vi "InitDrive.vi"   [LabVIEW 2018]
uses:
  <vilib>/Rock Robotics/WPI/ThirdParty/REV Robotics/SPARK MAX/Typedef/Spark MAX Idle Mode.ctl
  refnums.vi
  <vilib>/Rock Robotics/WPI/MotorControl/WPI_MotorControlOpen SPARK_MAX.vi
  <vilib>/Rock Robotics/SystemInterfaces/DIO/FPGA_DIOPWMChannel.ctl
types:
  T1 = typedef "Spark MAX Idle Mode.ctl" = enum16{"Coast", "Brake"}
  T2 = typedef "FPGA_DIOPWMChannel.ctl" = enum8{"PWM 0", "PWM 1", "PWM 2", "PWM 3", "PWM 4", "PWM 5", "PWM 6", "PWM 7", "PWM 8", "PWM 9", "PWM MXP 0", "PWM MXP 1", "PWM MXP 2", "PWM MXP 3", "PWM MXP 4", "PWM MXP 5", "PWM MXP 6", "PWM MXP 7", "PWM MXP 8", "PWM MXP 9", "Invalid"}
  T3 = typedef "WPI_MotorControlDeviceRef.ctl" = cluster{"DeviceStatus":errorcluster, "Type":T4, "PWM":cluster{"PWM Channel":T2, "DeadBand":T5}, "CAN":cluster{"Device Number":u8, "SetOutput VI Ref":variant, "GetOutput VI Ref":variant, "Enable VI Ref":variant, "Disable VI Ref":variant, "Data":variant}, "Invert":bool, "DIO PWM":cluster{"PWM \"Enable\" Channel":T2, "DIOChannel":T6, "PWM Rate":dbl}}
  T4 = typedef "WPI_MotorControlType.ctl" = enum16{"PWM", "CAN", "DIO PWM"}
  T5 = typedef "WPI_PWMDeadband.ctl" = cluster{"Name":string, "maxPositivePwm":i32, "minPositivePwm":i32, "centerPwm":i32, "maxNegativePwm":i32, "minNegativePwm":i32, "angularRange":u16}
  T6 = typedef "FPGA_DIOChannel.ctl" = enum8{"DIO 0", "DIO 1", "DIO 2", "DIO 3", "DIO 4", "DIO 5", "DIO 6", "DIO 7", "DIO 8", "DIO 9", "DIO MXP 0", "DIO MXP 1", "DIO MXP 2", "DIO MXP 3", "DIO MXP 4", "DIO MXP 5", "DIO MXP 6", "DIO MXP 7", "DIO MXP 8", "DIO MXP 9", "DIO MXP 10", "DIO MXP 11", "DIO MXP 12", "DIO MXP 13", "DIO MXP 14", "DIO MXP 15", "SPI Port CS1", "SPI Port CS2", "SPI Port CS3", "SPI Port MISO", "SPI Port MOSI", "Invalid"}
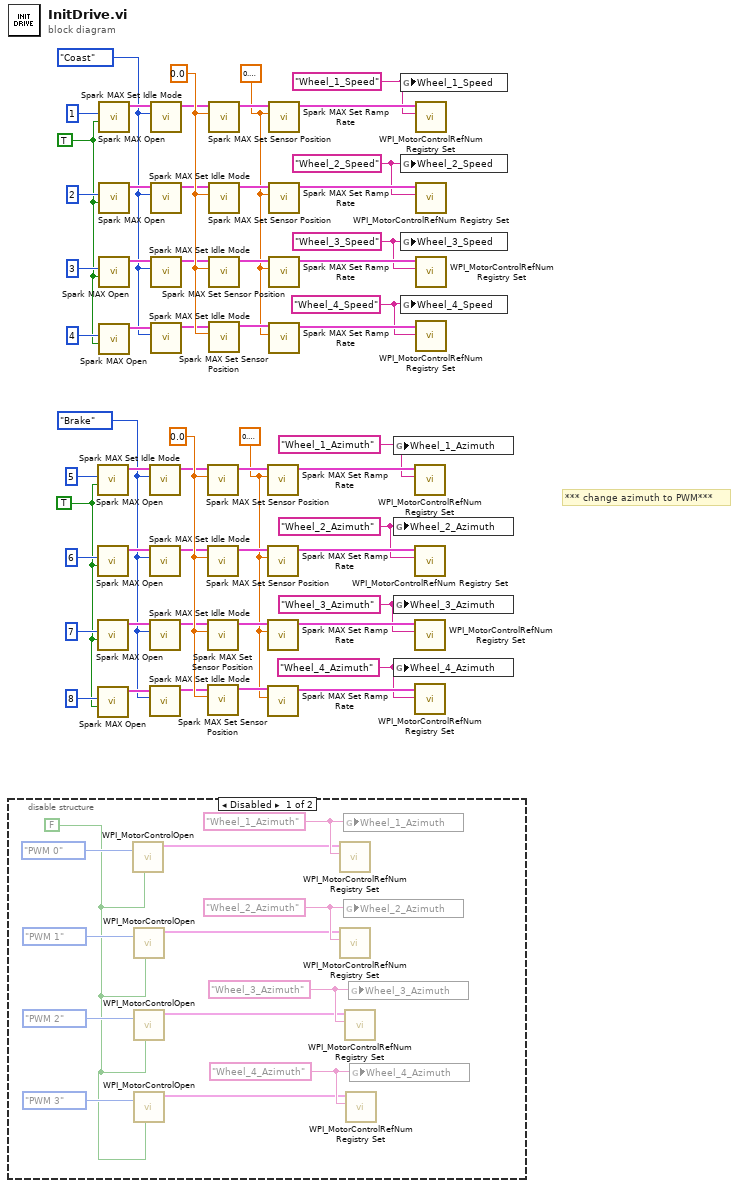
[diagram p0: block diagram]
diagram:
  w28 = 0.0
  w2 = TRUE
  w4 = "Wheel_3_Azimuth" ("refnum name")
  w3 = "Wheel_4_Azimuth" ("refnum name")
  w5 = "Wheel_2_Azimuth" ("refnum name")
  w1 = Spark_MAX_Idle_Mode."Brake" ("Idle Mode")
  w6 = "Wheel_1_Azimuth" ("refnum name")
  w7 = sgl 0.1 ("Seconds from neutral to full (0)")
  w56 = 0.0
  w30 = TRUE
  w32 = "Wheel_3_Speed" ("refnum name")
  w31 = "Wheel_4_Speed" ("refnum name")
  w33 = "Wheel_2_Speed" ("refnum name")
  w29 = Spark_MAX_Idle_Mode."Coast" ("Idle Mode")
  w34 = "Wheel_1_Speed" ("refnum name")
  w35 = sgl 0.2 ("Seconds from neutral to full (0)")
  # "*** change azimuth to PWM***"
  n1 = disable-structure shown="Disabled" {
    frame Disabled {
      w58 = "Wheel_4_Azimuth" ("refnum name")
      w60 = "Wheel_3_Azimuth" ("refnum name")
      w62 = "Wheel_2_Azimuth" ("refnum name")
      w64 = "Wheel_1_Azimuth" ("refnum name")
      w65 = FALSE ("Invert")
      n2 = call-poly <vilib>:"WPI_MotorControlOpen.vi"("Invert"=w65, "PWM Channel"=FPGA_DIOPWMChannel."PWM 0") -> ("MotorControlDeviceRef"=w63:T3)  [unwired: 8 in, 1 out]
      n3 = call-poly <vilib>:"WPI_MotorControlOpen.vi"("Invert"=w65, "PWM Channel"=FPGA_DIOPWMChannel."PWM 1") -> ("MotorControlDeviceRef"=w61:T3)  [unwired: 8 in, 1 out]
      n4 = call-poly <vilib>:"WPI_MotorControlOpen.vi"("Invert"=w65, "PWM Channel"=FPGA_DIOPWMChannel."PWM 2") -> ("MotorControlDeviceRef"=w59:T3)  [unwired: 8 in, 1 out]
      n5 = call-poly <vilib>:"WPI_MotorControlOpen.vi"("Invert"=w65, "PWM Channel"=FPGA_DIOPWMChannel."PWM 3") -> ("MotorControlDeviceRef"=w57:T3)  [unwired: 8 in, 1 out]
      n6 = call <vilib>:"WPI_MotorControlRefNum Registry Set.vi"("refnum name"=w64, "MotorControlDevRef"=w63) -> ()  [unwired: 8 in, 2 out]
      n7 = call <vilib>:"WPI_MotorControlRefNum Registry Set.vi"("refnum name"=w62, "MotorControlDevRef"=w61) -> ()  [unwired: 8 in, 2 out]
      n8 = global write "refnums.vi" "Wheel_1_Azimuth"(w64) -> ()
      n9 = global write "refnums.vi" "Wheel_2_Azimuth"(w62) -> ()
      n10 = call <vilib>:"WPI_MotorControlRefNum Registry Set.vi"("refnum name"=w60, "MotorControlDevRef"=w59) -> ()  [unwired: 8 in, 2 out]
      n11 = call <vilib>:"WPI_MotorControlRefNum Registry Set.vi"("refnum name"=w58, "MotorControlDevRef"=w57) -> ()  [unwired: 8 in, 2 out]
      n12 = global write "refnums.vi" "Wheel_3_Azimuth"(w60) -> ()
      n13 = global write "refnums.vi" "Wheel_4_Azimuth"(w58) -> ()
    }
    frame Enabled {
    }
  }
  n14 = call <vilib>:"Spark MAX Open.vi"("Invert"=w2, "Device Number"=u8 5 ("Drive 1R")) -> ("MotorControlDeviceRef"=w8:T3)  [unwired: 8 in, 1 out]
  n15 = call <vilib>:"Spark MAX Open.vi"("Invert"=w2, "Device Number"=u8 6 ("Drive 2R")) -> ("MotorControlDeviceRef"=w11:T3)  [unwired: 8 in, 1 out]
  n16 = call <vilib>:"Spark MAX Open.vi"("Invert"=w2, "Device Number"=u8 7 ("Drive  3R")) -> ("MotorControlDeviceRef"=w17:T3)  [unwired: 8 in, 1 out]
  n17 = call <vilib>:"Spark MAX Open.vi"("Invert"=w2, "Device Number"=u8 8 ("Drive 4L")) -> ("MotorControlDeviceRef"=w14:T3)  [unwired: 8 in, 1 out]
  n18 = call <vilib>:"Spark MAX Open.vi"("Invert"=w30, "Device Number"=u8 1 ("Drive 1R")) -> ("MotorControlDeviceRef"=w36:T3)  [unwired: 8 in, 1 out]
  n19 = call <vilib>:"Spark MAX Open.vi"("Invert"=w30, "Device Number"=u8 2 ("Drive 2R")) -> ("MotorControlDeviceRef"=w39:T3)  [unwired: 8 in, 1 out]
  n20 = call <vilib>:"Spark MAX Open.vi"("Invert"=w30, "Device Number"=u8 3 ("Drive  3R")) -> ("MotorControlDeviceRef"=w45:T3)  [unwired: 8 in, 1 out]
  n21 = call <vilib>:"Spark MAX Open.vi"("Invert"=w30, "Device Number"=u8 4 ("Drive 4L")) -> ("MotorControlDeviceRef"=w42:T3)  [unwired: 8 in, 1 out]
  n22 = call <vilib>:"Spark MAX Set Idle Mode.vi"("Idle Mode"=w1, "MotorControlDeviceRef in"=w8) -> ("MotorControlDeviceRef out"=w20:T3)  [unwired: 8 in, 1 out]
  n23 = call <vilib>:"Spark MAX Set Idle Mode.vi"("Idle Mode"=w1, "MotorControlDeviceRef in"=w11) -> ("MotorControlDeviceRef out"=w22:T3)  [unwired: 8 in, 1 out]
  n24 = call <vilib>:"Spark MAX Set Idle Mode.vi"("Idle Mode"=w1, "MotorControlDeviceRef in"=w17) -> ("MotorControlDeviceRef out"=w24:T3)  [unwired: 8 in, 1 out]
  n25 = call <vilib>:"Spark MAX Set Idle Mode.vi"("Idle Mode"=w1, "MotorControlDeviceRef in"=w14) -> ("MotorControlDeviceRef out"=w26:T3)  [unwired: 8 in, 1 out]
  n26 = call <vilib>:"Spark MAX Set Idle Mode.vi"("Idle Mode"=w29, "MotorControlDeviceRef in"=w36) -> ("MotorControlDeviceRef out"=w48:T3)  [unwired: 8 in, 1 out]
  n27 = call <vilib>:"Spark MAX Set Idle Mode.vi"("Idle Mode"=w29, "MotorControlDeviceRef in"=w39) -> ("MotorControlDeviceRef out"=w50:T3)  [unwired: 8 in, 1 out]
  n28 = call <vilib>:"Spark MAX Set Idle Mode.vi"("Idle Mode"=w29, "MotorControlDeviceRef in"=w45) -> ("MotorControlDeviceRef out"=w52:T3)  [unwired: 8 in, 1 out]
  n29 = call <vilib>:"Spark MAX Set Idle Mode.vi"("Idle Mode"=w29, "MotorControlDeviceRef in"=w42) -> ("MotorControlDeviceRef out"=w54:T3)  [unwired: 8 in, 1 out]
  n30 = call <vilib>:"Spark MAX Set Sensor Position.vi"("Position"=w28, "MotorControlDeviceRef"=w20) -> ("MotorControlDeviceRef"=w21:T3)  [unwired: 8 in, 1 out]
  n31 = call <vilib>:"Spark MAX Set Sensor Position.vi"("Position"=w28, "MotorControlDeviceRef"=w22) -> ("MotorControlDeviceRef"=w23:T3)  [unwired: 8 in, 1 out]
  n32 = call <vilib>:"Spark MAX Set Sensor Position.vi"("Position"=w28, "MotorControlDeviceRef"=w24) -> ("MotorControlDeviceRef"=w25:T3)  [unwired: 8 in, 1 out]
  n33 = call <vilib>:"Spark MAX Set Sensor Position.vi"("Position"=w28, "MotorControlDeviceRef"=w26) -> ("MotorControlDeviceRef"=w27:T3)  [unwired: 8 in, 1 out]
  n34 = call <vilib>:"Spark MAX Set Sensor Position.vi"("Position"=w56, "MotorControlDeviceRef"=w48) -> ("MotorControlDeviceRef"=w49:T3)  [unwired: 8 in, 1 out]
  n35 = call <vilib>:"Spark MAX Set Sensor Position.vi"("Position"=w56, "MotorControlDeviceRef"=w50) -> ("MotorControlDeviceRef"=w51:T3)  [unwired: 8 in, 1 out]
  n36 = call <vilib>:"Spark MAX Set Sensor Position.vi"("Position"=w56, "MotorControlDeviceRef"=w52) -> ("MotorControlDeviceRef"=w53:T3)  [unwired: 8 in, 1 out]
  n37 = call <vilib>:"Spark MAX Set Sensor Position.vi"("Position"=w56, "MotorControlDeviceRef"=w54) -> ("MotorControlDeviceRef"=w55:T3)  [unwired: 8 in, 1 out]
  n38 = call <vilib>:"Spark MAX Set Ramp Rate.vi"("Seconds from neutral to full (0)"=w7, "MotorControlDeviceRef in"=w21) -> ("MotorControlDeviceRef"=w9:T3)  [unwired: 8 in, 1 out]
  n39 = call <vilib>:"Spark MAX Set Ramp Rate.vi"("Seconds from neutral to full (0)"=w7, "MotorControlDeviceRef in"=w23) -> ("MotorControlDeviceRef"=w13:T3)  [unwired: 8 in, 1 out]
  n40 = call <vilib>:"Spark MAX Set Ramp Rate.vi"("Seconds from neutral to full (0)"=w7, "MotorControlDeviceRef in"=w25) -> ("MotorControlDeviceRef"=w19:T3)  [unwired: 8 in, 1 out]
  n41 = call <vilib>:"Spark MAX Set Ramp Rate.vi"("Seconds from neutral to full (0)"=w7, "MotorControlDeviceRef in"=w27) -> ("MotorControlDeviceRef"=w16:T3)  [unwired: 8 in, 1 out]
  n42 = call <vilib>:"Spark MAX Set Ramp Rate.vi"("Seconds from neutral to full (0)"=w35, "MotorControlDeviceRef in"=w49) -> ("MotorControlDeviceRef"=w37:T3)  [unwired: 8 in, 1 out]
  n43 = call <vilib>:"Spark MAX Set Ramp Rate.vi"("Seconds from neutral to full (0)"=w35, "MotorControlDeviceRef in"=w51) -> ("MotorControlDeviceRef"=w41:T3)  [unwired: 8 in, 1 out]
  n44 = call <vilib>:"Spark MAX Set Ramp Rate.vi"("Seconds from neutral to full (0)"=w35, "MotorControlDeviceRef in"=w53) -> ("MotorControlDeviceRef"=w47:T3)  [unwired: 8 in, 1 out]
  n45 = call <vilib>:"Spark MAX Set Ramp Rate.vi"("Seconds from neutral to full (0)"=w35, "MotorControlDeviceRef in"=w55) -> ("MotorControlDeviceRef"=w44:T3)  [unwired: 8 in, 1 out]
  n46 = global write "refnums.vi" "Wheel_1_Azimuth"(w6) -> ()
  n47 = global write "refnums.vi" "Wheel_2_Azimuth"(w5) -> ()
  n48 = global write "refnums.vi" "Wheel_3_Azimuth"(w4) -> ()
  n49 = global write "refnums.vi" "Wheel_4_Azimuth"(w3) -> ()
  n50 = global write "refnums.vi" "Wheel_1_Speed"(w34) -> ()
  n51 = global write "refnums.vi" "Wheel_2_Speed"(w33) -> ()
  n52 = global write "refnums.vi" "Wheel_3_Speed"(w32) -> ()
  n53 = global write "refnums.vi" "Wheel_4_Speed"(w31) -> ()
  n54 = call <vilib>:"WPI_MotorControlRefNum Registry Set.vi"("refnum name"=w6, "MotorControlDevRef"=w9) -> ()  [unwired: 8 in, 2 out]
  n55 = call <vilib>:"WPI_MotorControlRefNum Registry Set.vi"("refnum name"=w5, "MotorControlDevRef"=w13) -> ()  [unwired: 8 in, 2 out]
  n56 = call <vilib>:"WPI_MotorControlRefNum Registry Set.vi"("refnum name"=w4, "MotorControlDevRef"=w19) -> ()  [unwired: 8 in, 2 out]
  n57 = call <vilib>:"WPI_MotorControlRefNum Registry Set.vi"("refnum name"=w3, "MotorControlDevRef"=w16) -> ()  [unwired: 8 in, 2 out]
  n58 = call <vilib>:"WPI_MotorControlRefNum Registry Set.vi"("refnum name"=w34, "MotorControlDevRef"=w37) -> ()  [unwired: 8 in, 2 out]
  n59 = call <vilib>:"WPI_MotorControlRefNum Registry Set.vi"("refnum name"=w33, "MotorControlDevRef"=w41) -> ()  [unwired: 8 in, 2 out]
  n60 = call <vilib>:"WPI_MotorControlRefNum Registry Set.vi"("refnum name"=w32, "MotorControlDevRef"=w47) -> ()  [unwired: 8 in, 2 out]
  n61 = call <vilib>:"WPI_MotorControlRefNum Registry Set.vi"("refnum name"=w31, "MotorControlDevRef"=w44) -> ()  [unwired: 8 in, 2 out]
